vi "dfd_Match Single Zeros and Poles.vi"(10 "real poles":cdb[](array[numeric]), 11 "real zeros":cdb[](array[numeric])) -> (1 "matched z&p":cluster{"zeros":cdb[], "poles":cdb[]}[](array[cluster]), 2 "remaining poles":cdb[](array[numeric]), 3 "remaining zeros":cdb[](array[numeric]))   [LabVIEW 2017, in "NI_DigFilterLicensed.lvlib"]
uses:
  <vilib>/addons/Digital Filter Design/NI_DigFilterLicensed.lvlib
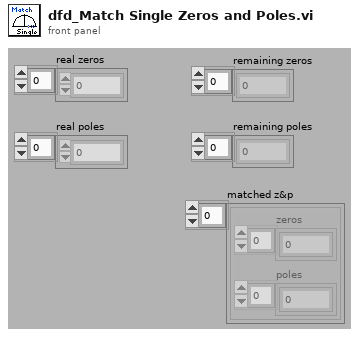
[diagram p1: front panel]
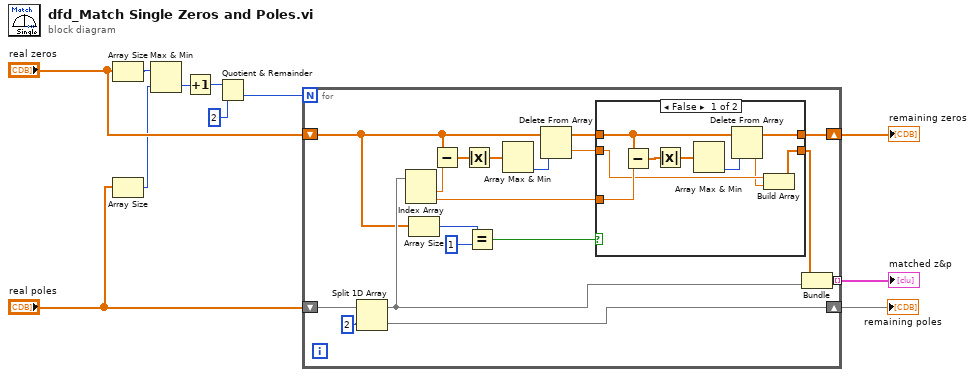
[diagram p0: block diagram]
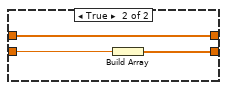
[diagram p2: hidden frame]
diagram:
  n1 = Array Size(array="real zeros") -> (size(s)=w2:i32)
  n2 = Array Size(array="real poles") -> (size(s)=w3:i32)
  n3 = Max & Min(x=w2, y=w3) -> (min(x,y)=w1:i32)  [unwired: 1 out]
  n4 = Increment(x=w1) -> (x+1=w7:i32)
  n5 = Quotient & Remainder(x=w7, y=2) -> (floor(x/y)=w4:i32)  [unwired: 1 out]
  n6 = for {
    N: w4 -> [_]
    shift-right: [w17] -> w11
    shift-left: "real zeros" -> [w12]
    shift-right: [w25] -> w10
    shift-left: "real poles" -> [w27]
    tunnel: [w13] -> w5 mode=indexing
    n7 = Split 1D Array(array=w27, index=2) -> (first subarray=w23:cdb[], second subarray=w25:cdb[])
    n8 = Index Array(array=w23) -> (element #1=w24:cdb, element #2=w15:cdb)  [unwired: 2 in]
    n9 = Array Size(array=w12) -> (size(s)=w21:i32)
    n10 = Subtract(x=w12, y=w24) -> (x-y=w29:cdb[])
    n11 = Absolute Value(x=w29) -> (abs(x)=w28:dbl[])
    n12 = Equal?(x=w21, y=1) -> (x = y?=w18:bool)
    n13 = Array Max & Min(array=w28) -> (min index (indices)=w22:i32)  [unwired: 3 out]
    n14 = Delete From Array(array=w12, index=w22) -> (deleted portion=w16:cdb, array with subset deleted=w19:cdb[])  [unwired: 1 in]
    n15 = case shown="False" w18 {
      tunnel: w19 -> [w35 w41]
      tunnel: [w33 w41] -> w17
      tunnel: w16 -> [w32 w40]
      tunnel: [w30 w39] -> w14
      tunnel: w15 -> [w34 _]
      frame False {
        n16 = Subtract(x=w35, y=w34) -> (x-y=w36:cdb[])
        n17 = Absolute Value(x=w36) -> (abs(x)=w37:dbl[])
        n18 = Array Max & Min(array=w37) -> (min index (indices)=w38:i32)  [unwired: 3 out]
        n19 = Delete From Array(array=w35, index=w38) -> (deleted portion=w31:cdb, array with subset deleted=w33:cdb[])  [unwired: 1 in]
        n20 = Build Array(w32, w31) -> (w30:cdb[])
      }
      frame True {
        n21 = Build Array(w40) -> (w39:cdb[])
      }
    }
    n22 = Bundle(w14, w23) -> (w13:cluster{cdb[], cdb[]})  [unwired: 1 out]
  }
  "remaining zeros" <- w11
  "remaining poles" <- w10
  "matched z&p" <- w5
